vi "command_mem.vi"(0 "input":T1, 1 "WR":T3, 2 "R_ip":bool, 3 "R":bool, 4 "С":bool) -> (5 "test":bool, 6 "output":T2)   [LabVIEW 2013]
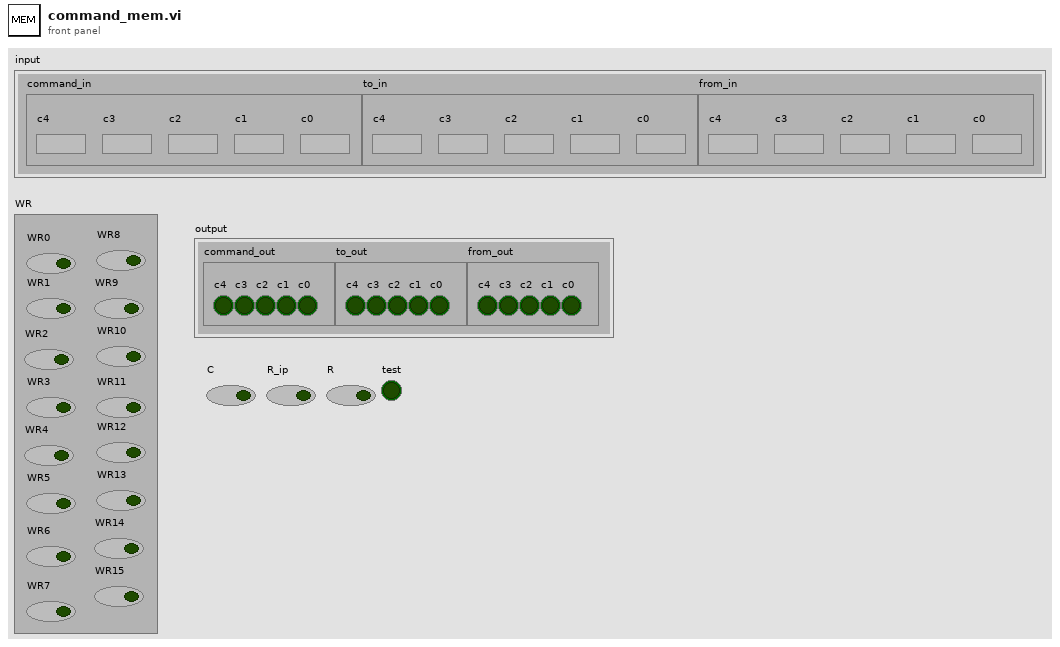
[diagram p1: front panel]
types:
  T1 = cluster{"command_in":cluster{"c4":bool, "c3":bool, "c2":bool, "c1":bool, "c0":bool}, "to_in":cluster{"c4":bool, "c3":bool, "c2":bool, "c1":bool, "c0":bool}, "from_in":cluster{"c4":bool, "c3":bool, "c2":bool, "c1":bool, "c0":bool}}
  T2 = cluster{"command_out":cluster{"c4":bool, "c3":bool, "c2":bool, "c1":bool, "c0":bool}, "to_out":cluster{"c4":bool, "c3":bool, "c2":bool, "c1":bool, "c0":bool}, "from_out":cluster{"c4":bool, "c3":bool, "c2":bool, "c1":bool, "c0":bool}}
  T3 = cluster{"WR0":bool, "WR1":bool, "WR2":bool, "WR3":bool, "WR4":bool, "WR5":bool, "WR6":bool, "WR7":bool, "WR8":bool, "WR9":bool, "WR10":bool, "WR11":bool, "WR12":bool, "WR13":bool, "WR14":bool, "WR15":bool}
  T4 = cluster{"q0":bool, "q1":bool, "q2":bool, "q3":bool, "q4":bool, "q5":bool, "q6":bool, "q7":bool, "p8":bool, "p9":bool, "p10":bool, "p11":bool, "p12":bool, "p13":bool, "p14":bool, "p15":bool}
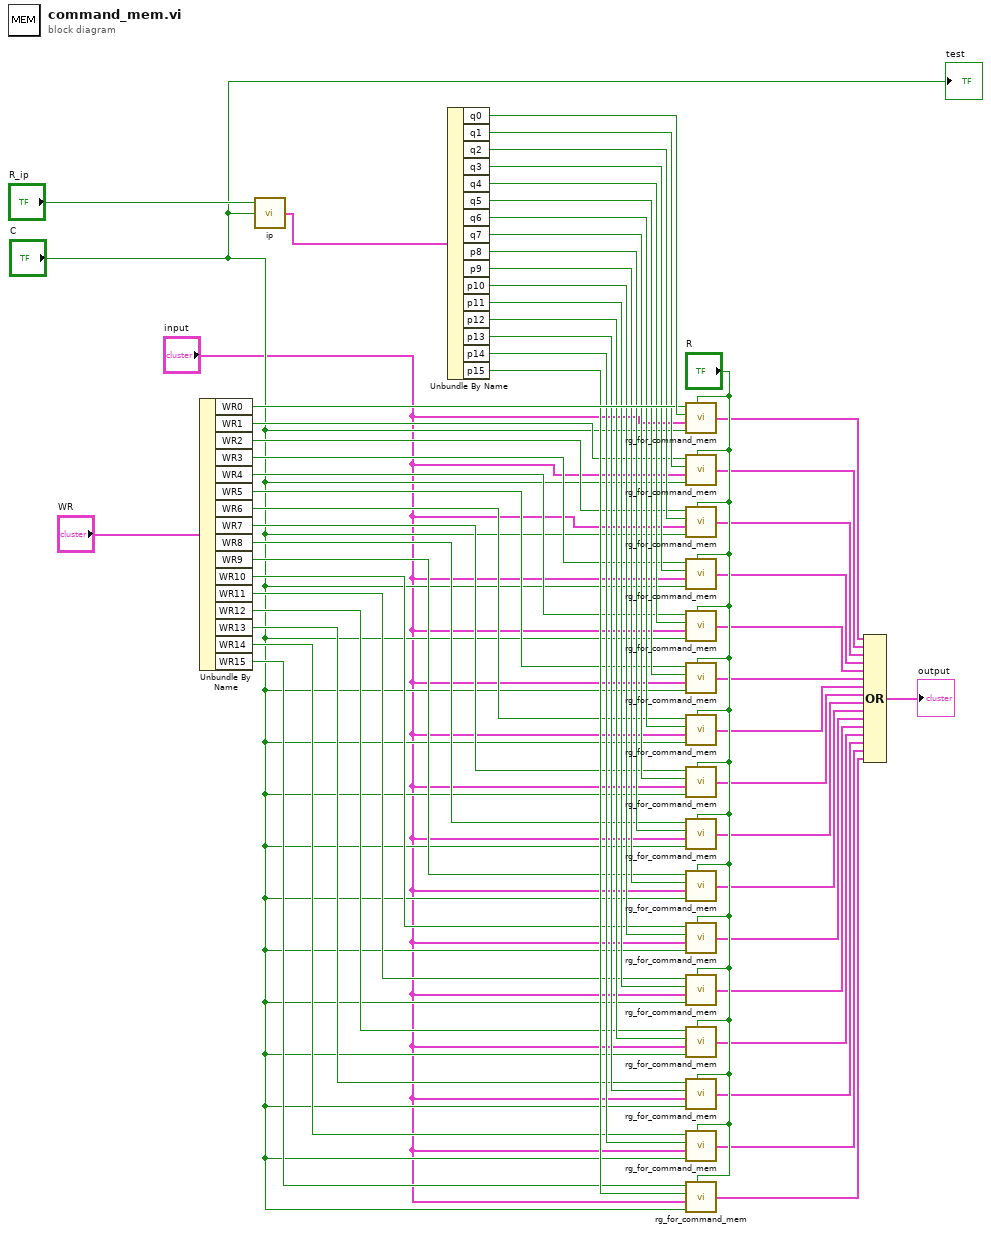
[diagram p0: block diagram]
diagram:
  n1 = Unbundle By Name("WR") -> ("WR0"=w51:bool, "WR1"=w34:bool, "WR2"=w33:bool, "WR3"=w32:bool, "WR4"=w31:bool, "WR5"=w30:bool, "WR6"=w29:bool, "WR7"=w28:bool, "WR8"=w27:bool, "WR9"=w26:bool, "WR10"=w25:bool, "WR11"=w24:bool, "WR12"=w23:bool, "WR13"=w22:bool, "WR14"=w21:bool, "WR15"=w20:bool)
  n2 = call "ip.vi"("T"="С", "R"="R_ip") -> ("com_number"=w54:T4)  [unwired: 1 in]
  n3 = Unbundle By Name(w54) -> ("q0"=w52:bool, "q1"=w50:bool, "q2"=w49:bool, "q3"=w48:bool, "q4"=w47:bool, "q5"=w46:bool, "q6"=w45:bool, "q7"=w44:bool, "p8"=w43:bool, "p9"=w42:bool, "p10"=w41:bool, "p11"=w40:bool, "p12"=w39:bool, "p13"=w38:bool, "p14"=w36:bool, "p15"=w35:bool)
  n4 = call "rg_for_command_mem.vi"("WR"=w51, "RD"=w52, "input"="input", "такты"="С", "R"="R") -> ("output"=w18:T2)
  n5 = call "rg_for_command_mem.vi"("WR"=w34, "RD"=w50, "input"="input", "такты"="С", "R"="R") -> ("output"=w17:T2)
  n6 = call "rg_for_command_mem.vi"("WR"=w33, "RD"=w49, "input"="input", "такты"="С", "R"="R") -> ("output"=w16:T2)
  n7 = call "rg_for_command_mem.vi"("WR"=w32, "RD"=w48, "input"="input", "такты"="С", "R"="R") -> ("output"=w15:T2)
  n8 = call "rg_for_command_mem.vi"("WR"=w31, "RD"=w47, "input"="input", "такты"="С", "R"="R") -> ("output"=w14:T2)
  n9 = call "rg_for_command_mem.vi"("WR"=w30, "RD"=w46, "input"="input", "такты"="С", "R"="R") -> ("output"=w13:T2)
  n10 = call "rg_for_command_mem.vi"("WR"=w29, "RD"=w45, "input"="input", "такты"="С", "R"="R") -> ("output"=w2:T2)
  n11 = call "rg_for_command_mem.vi"("WR"=w28, "RD"=w44, "input"="input", "такты"="С", "R"="R") -> ("output"=w3:T2)
  n12 = call "rg_for_command_mem.vi"("WR"=w27, "RD"=w43, "input"="input", "такты"="С", "R"="R") -> ("output"=w4:T2)
  n13 = call "rg_for_command_mem.vi"("WR"=w26, "RD"=w42, "input"="input", "такты"="С", "R"="R") -> ("output"=w5:T2)
  n14 = call "rg_for_command_mem.vi"("WR"=w25, "RD"=w41, "input"="input", "такты"="С", "R"="R") -> ("output"=w6:T2)
  n15 = call "rg_for_command_mem.vi"("WR"=w24, "RD"=w40, "input"="input", "такты"="С", "R"="R") -> ("output"=w7:T2)
  n16 = call "rg_for_command_mem.vi"("WR"=w23, "RD"=w39, "input"="input", "такты"="С", "R"="R") -> ("output"=w8:T2)
  n17 = call "rg_for_command_mem.vi"("WR"=w22, "RD"=w38, "input"="input", "такты"="С", "R"="R") -> ("output"=w9:T2)
  n18 = call "rg_for_command_mem.vi"("WR"=w21, "RD"=w36, "input"="input", "такты"="С", "R"="R") -> ("output"=w10:T2)
  n19 = call "rg_for_command_mem.vi"("WR"=w20, "RD"=w35, "input"="input", "такты"="С", "R"="R") -> ("output"=w12:T2)
  n20 = Compound Arithmetic op=OR(w18, w17, w16, w15, w14, w13, w2, w3, w4, w5, w6, w7, w8, w9, w10, w12) -> (→"output":T2)
  "test" <- "С"
